vi "Close SLM.vi"(11 "Boolean":bool=TRUE) -> (3 "Boolean 2":bool=TRUE)   [LabVIEW 2014]
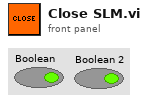
[diagram p1: front panel]
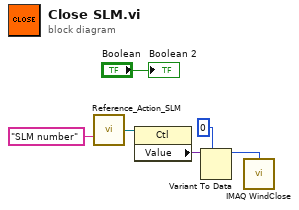
[diagram p0: block diagram]
diagram:
  n1 = call "Reference_Action_SLM.vi"("Control Name"="SLM number") -> ("Ref OUT"=w3:refnum<vi>)  [unwired: 12 in, 2 out]
  n2 = property class="Ctl"(reference=w3) -> ("Value"=w4:variant)  [unwired: 1 in, 2 out]
  n3 = Variant To Data(type=0, Variant=w4) -> (data=w1:i32)  [unwired: 1 in, 1 out]
  n4 = call "IMAQ WindClose"("Window Number (0...15)"=w1) -> ()  [unwired: 2 in, 4 out]
  "Boolean 2" <- "Boolean"
